vi "0926New Project.vi"() -> ()   [LabVIEW 2011] (continued)
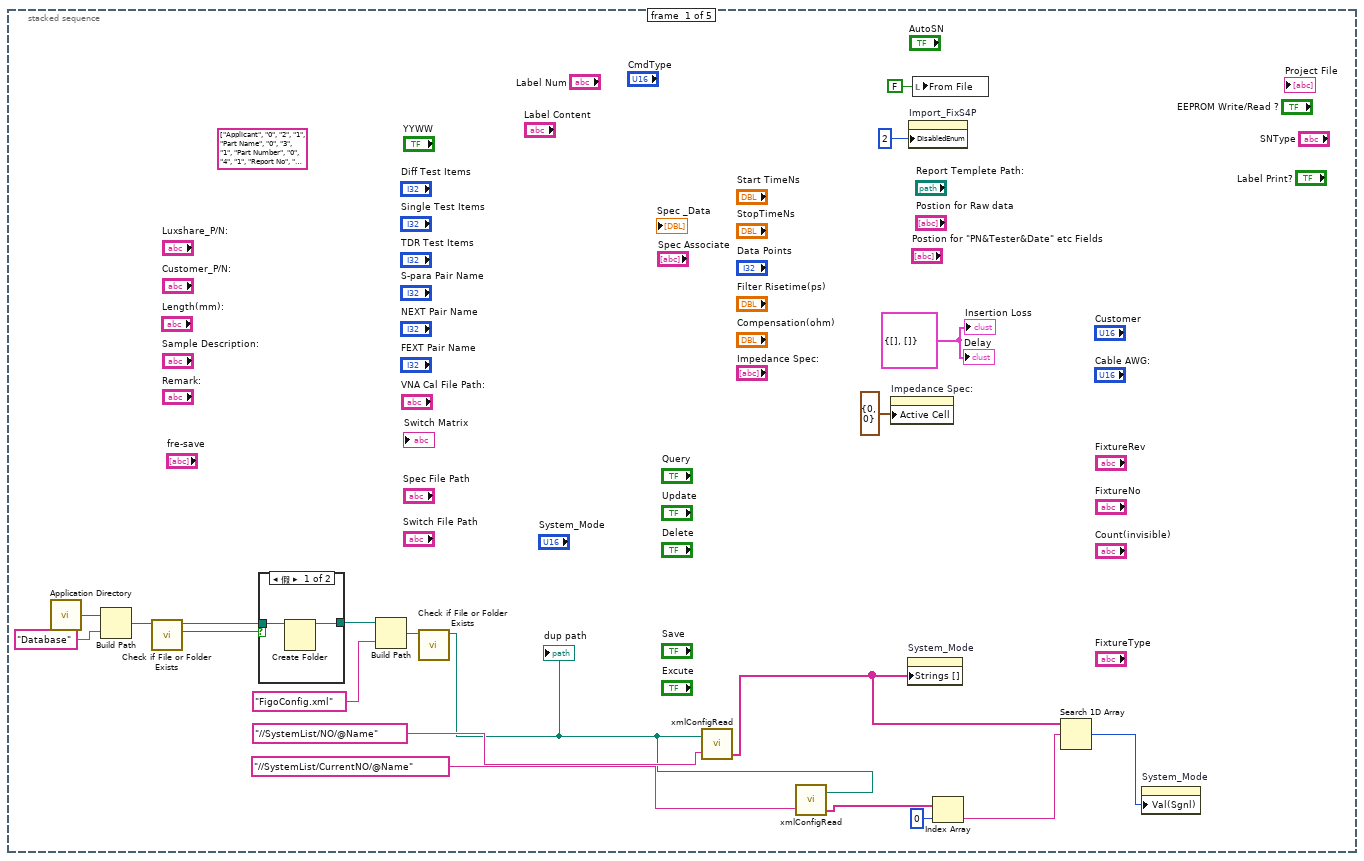
[diagram p3: hidden frame]
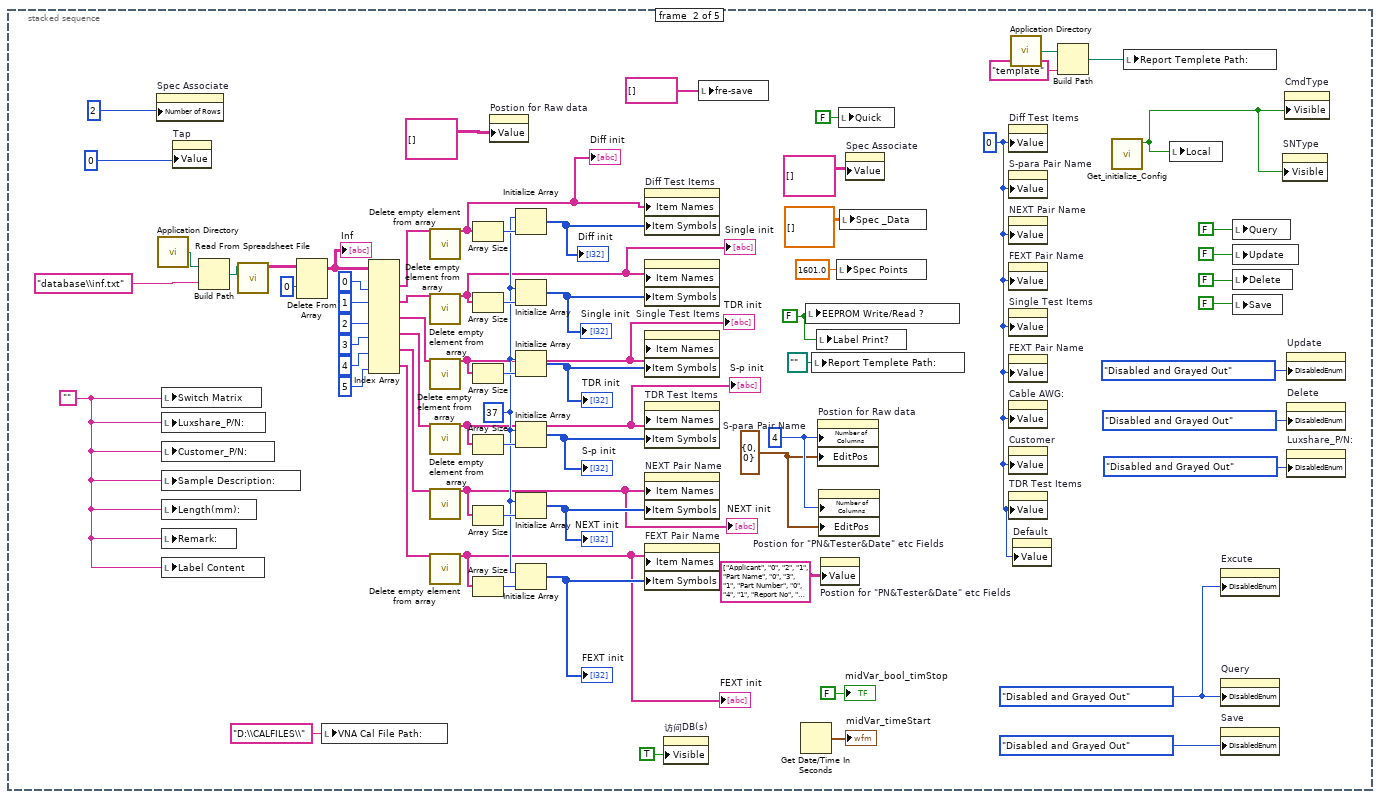
[diagram p5: hidden frame]
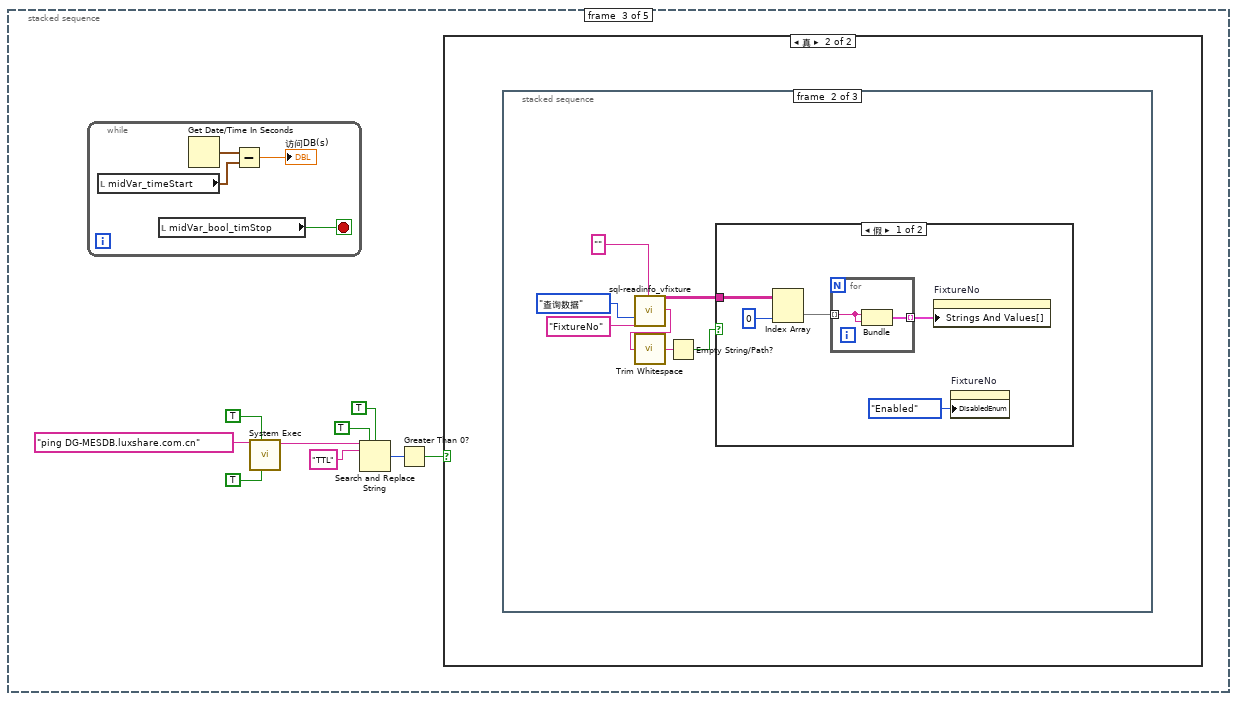
[diagram p6: hidden frame]
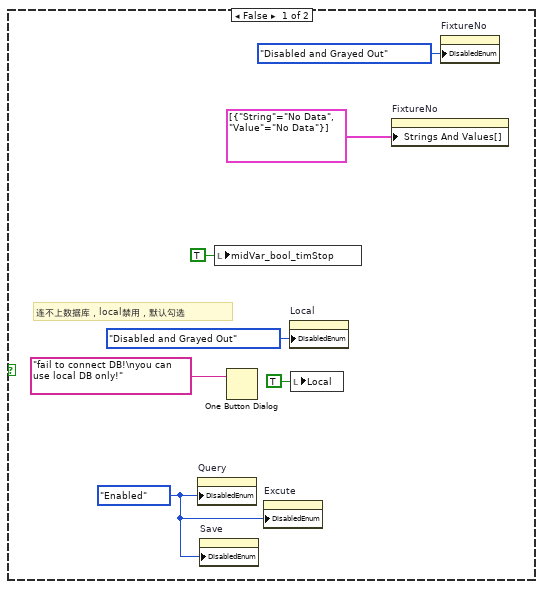
[diagram p7: hidden frame]
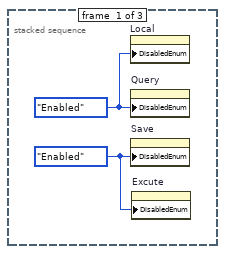
[diagram p8: hidden frame]
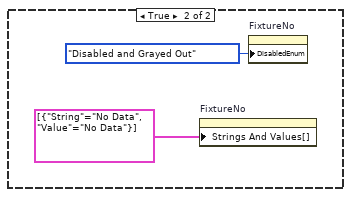
[diagram p9: hidden frame]
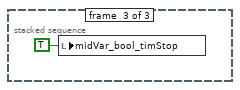
[diagram p10: hidden frame]
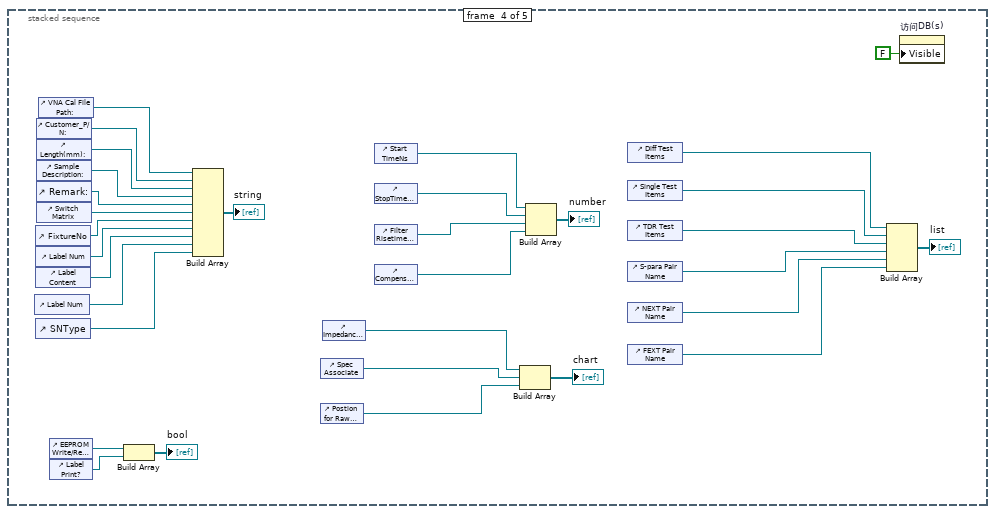
[diagram p11: hidden frame]
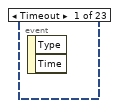
[diagram p12: hidden frame]
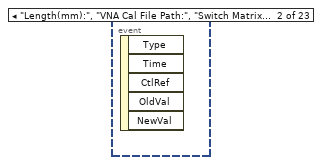
[diagram p13: hidden frame]
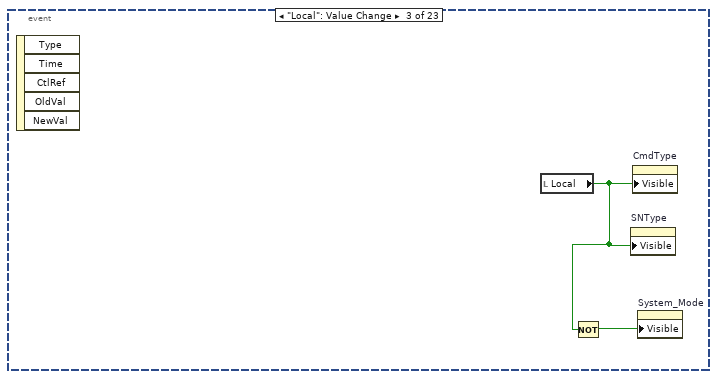
[diagram p14: hidden frame]
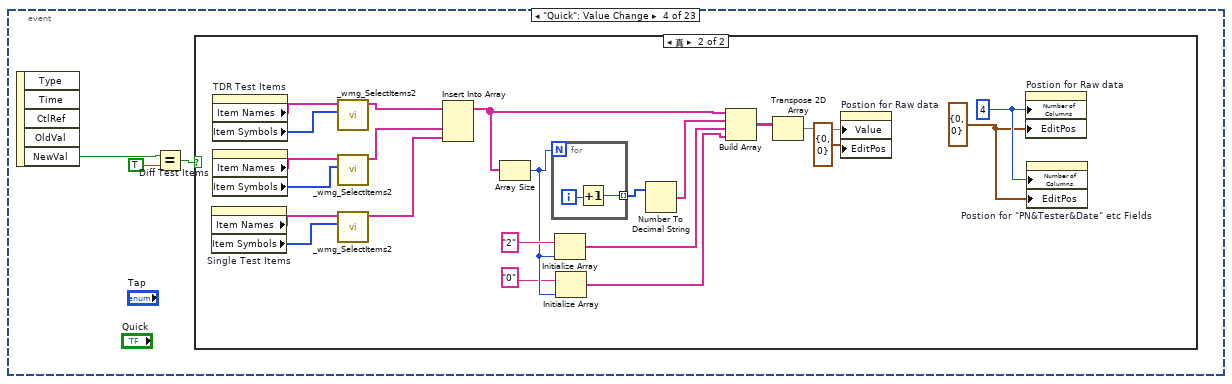
[diagram p15: hidden frame]
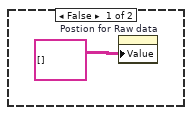
[diagram p16: hidden frame]
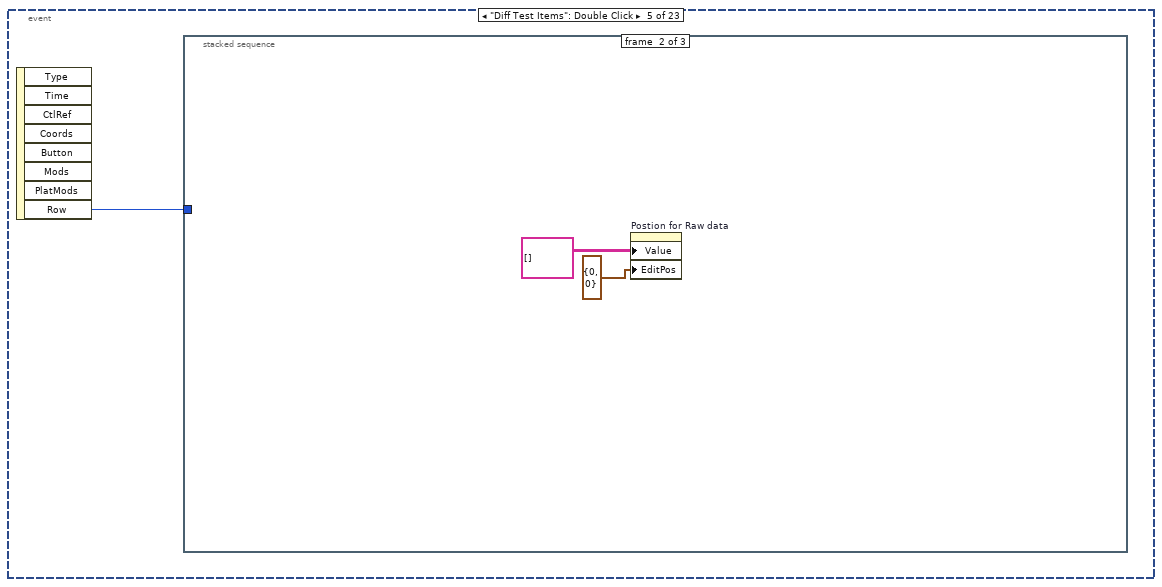
[diagram p17: hidden frame]
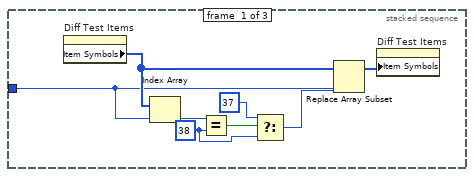
[diagram p18: hidden frame]
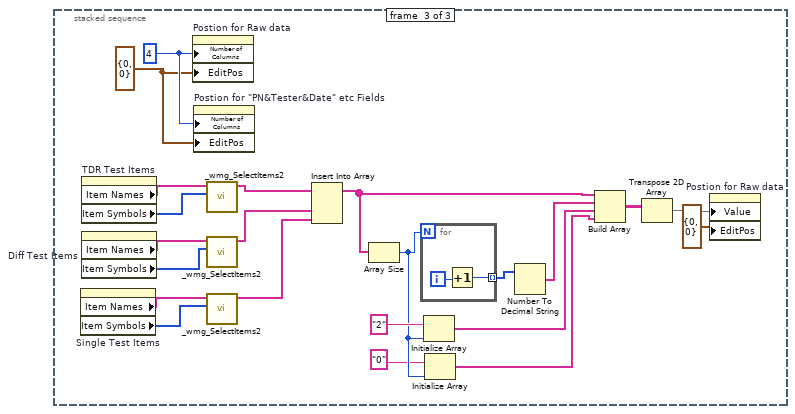
[diagram p19: hidden frame]
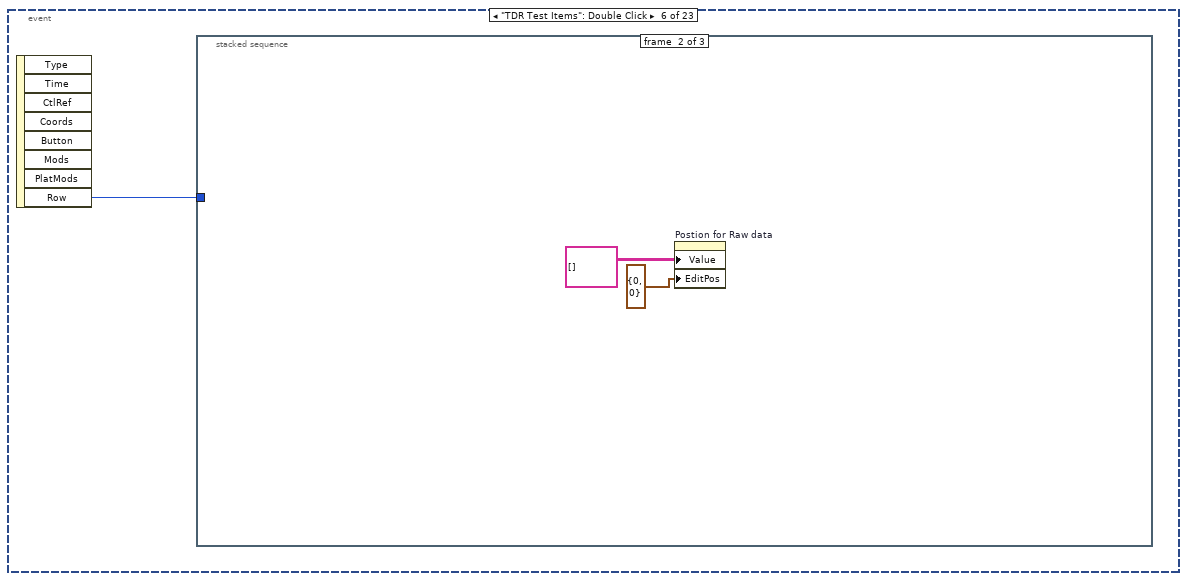
[diagram p20: hidden frame]
                    n969 = Number To Decimal String(number=w1171) -> (decimal integer string=w1169:string)  [unwired: 1 in]
                    n970 = call "impedance spec.vi"("Impedance Spec:"=w1168) -> ("Impedance spec string"=w1167:string)  [unwired: 10 in]
                    n971 = call <vilib>:"Trim Whitespace.vi"("string"=w1152) -> ("trimmed string"=w1144:string)  [unwired: 1 in]
                    n972 = Build Array(w1149, w1148, w1147, w1146, w1145, w1169, w1167, w1150, w1151, w1144) -> (→"TDR Setting":string[])
                    n973 = local read "Report Templete Path:"() -> (w1153:path)
                    n974 = property on="Postion for Raw data" class="Tbl (严格)"() -> ("Value"=w1165:string[][])  [unwired: 2 in, 2 out]
                    n975 = property on="Postion for \"PN&Tester&Date\" etc Fields" class="Tbl (严格)"() -> ("Value"=w1164:string[][])  [unwired: 2 in, 2 out]
                    n976 = Array To Spreadsheet String(array=w1165, 3:w1166) -> (spreadsheet string=w1161:string)  [unwired: 1 in]
                    n977 = Array To Spreadsheet String(array=w1164, 3:w1166) -> (spreadsheet string=w1159:string)  [unwired: 1 in]
                    n978 = Path To String(path=w1153) -> (string=w1154:string)
                    n979 = Search and Replace String(replace all?=TRUE ("替换全部？(F)"), input string=w1161, search string=w1156, replace string=w1155) -> (result string=w1158:string)  [unwired: 4 in, 3 out]
                    n980 = Search and Replace String(replace all?=TRUE ("替换全部？(F)"), input string=w1159, search string=w1156, replace string=w1155) -> (result string=w1157:string)  [unwired: 4 in, 3 out]
                    n981 = Build Array(w1154, w1158, w1157) -> (→"Report Config":string[])
                  }
                  frame #1 {
                    n982 = property on="S-para Pair Name" class="LstBox (严格)"() -> ("Item Names"=w1206:string[], "Item Symbols"=w1205:i32[])  [unwired: 2 in, 2 out]
                    n983 = property on="NEXT Pair Name" class="LstBox (严格)"() -> ("Item Names"=w1204:string[], "Item Symbols"=w1203:i32[])  [unwired: 2 in, 2 out]
                    n984 = property on="FEXT Pair Name" class="LstBox (严格)"() -> ("Item Names"=w1202:string[], "Item Symbols"=w1201:i32[])  [unwired: 2 in, 2 out]
                    n985 = local read "Spec Associate"() -> (w1195:string[][])
                    n986 = property on="Single Test Items" class="LstBox (严格)"() -> ("Item Names"=w1208:string[], "Item Symbols"=w1207:i32[])  [unwired: 2 in, 2 out]
                    n987 = property on="Diff Test Items" class="LstBox (严格)"() -> ("Item Names"=w1210:string[], "Item Symbols"=w1209:i32[])  [unwired: 2 in, 2 out]
                    n988 = property on="TDR Test Items" class="LstBox (严格)"() -> ("Item Names"=w1184:string[], "Item Symbols"=w1183:i32[])  [unwired: 2 in, 2 out]
                    n989 = call "Selected items.vi"("Item Syms"=w1205, "Item name"=w1206) -> ("Selected tem"=w1200:string[])  [unwired: 7 in, 2 out]
                    n990 = call "Selected items.vi"("Item Syms"=w1203, "Item name"=w1204) -> ("Selected tem"=w1199:string[])  [unwired: 7 in, 2 out]
                    n991 = call "Selected items.vi"("Item Syms"=w1201, "Item name"=w1202) -> ("Selected tem"=w1198:string[])  [unwired: 7 in, 2 out]
                    n992 = call "Selected items.vi"("Item Syms"=w1209, "Item name"=w1210) -> ("Selected tem"=w1197:string[])  [unwired: 7 in, 2 out]
                    n993 = call "Selected items.vi"("Item Syms"=w1207, "Item name"=w1208) -> ("Selected tem"=w1196:string[])  [unwired: 7 in, 2 out]
                    n994 = call "Selected items.vi"("Item Syms"=w1183, "Item name"=w1184) -> ("Selected tem"=w1181:string[])  [unwired: 7 in, 2 out]
                    n995 = Index Array(array=w1195, index (row)=1 ("索引 (行)")) -> (element=w1182:string[])  [unwired: 1 in]
                    n996 = local read "cancel dem2X?"() -> (w1176:bool)
                    n997 = local read "VNA Cal File Path:"() -> (w1178:string)
                    n998 = Select(t="TRUE", s=w1176, f="FALSE") -> (s? t:f=w1173:string)
                    n999 = local read "Report Config"() -> (w1179:string[])
                    n1000 = local read "TDR Setting"() -> (w1180:string[])
                    n1001 = Build Array(w1178) -> (w1193:string[])
                    n1002 = Number To Decimal String(number="ILD Spec") -> (decimal integer string=w1186:string)  [unwired: 1 in]
                    n1003 = Build Array(w1186) -> (w1185:string[])
                    n1004 = Build Array(w1173) -> (w1177:string[])
                    n1005 = Build Array(w1200, w1199, w1198, w1197, w1196, w1181, w1182, w1193, w1179, w1185, w1180, w1177) -> (w1192:string[][])
                    n1006 = Transpose 2D Array(2D array=w1192) -> (transposed array=w1191:string[][])
                    n1007 = Array To Spreadsheet String(delimiter (Tab)="#" ("分隔符(Tab)"), array=w1191, 3:"%s" ("格式字符串")) -> (spreadsheet string=→"Project Information":string)
                  }
                  frame #2 {
                    n1008 = local read "VNA Cal File Path:"() -> (w1230:string)
                    n1009 = property on="Diff Test Items" class="LstBox (严格)"() -> ("Item Symbols"=w1227:i32[])  [unwired: 2 in, 2 out]
                    n1010 = property on="Single Test Items" class="LstBox (严格)"() -> ("Item Symbols"=w1226:i32[])  [unwired: 2 in, 2 out]
                    n1011 = property on="TDR Test Items" class="LstBox (严格)"() -> ("Item Symbols"=w1225:i32[])  [unwired: 2 in, 2 out]
                    n1012 = property on="S-para Pair Name" class="LstBox (严格)"() -> ("Item Symbols"=w1224:i32[])  [unwired: 2 in, 2 out]
                    n1013 = property on="NEXT Pair Name" class="LstBox (严格)"() -> ("Item Symbols"=w1223:i32[])  [unwired: 2 in, 2 out]
                    n1014 = property on="FEXT Pair Name" class="LstBox (严格)"() -> ("Item Symbols"=w1219:i32[])  [unwired: 2 in, 2 out]
                    n1015 = local read "Luxshare_P/N:"() -> (w1217:string)
                    n1016 = local read "Length(mm):"() -> (w1231:string)
                    n1017 = String Length(string=w1217) -> (length=w1218:i32)
                    n1018 = Empty String/Path?(string/path=w1230) -> (empty?=w1228:bool)
                    n1019 = Empty String/Path?(string/path=w1231) -> (empty?=w1229:bool)
                    n1020 = Build Array(w1227, w1226, w1225, w1224, w1223, w1219) -> (w1222:i32[][])
                    n1021 = Not(x=w1229) -> (.not. x?=w1221:bool)
                    n1022 = Not(x=w1228) -> (.not. x?=w1220:bool)
                    n1023 = Greater Than 0?(x=w1218) -> (x > 0?=w1216:bool)
                    n1024 = call "_wmg_whetherItemsEmpty.vi"("Input"=w1222) -> ("bool"=w1232:bool)
                    n1025 = local read "Spec _Data"() -> (w1213:dbl[][])
                    n1026 = Compound Arithmetic op=AND(w1216, w1221, w1220, w1232) -> (→"save?":bool)
                    n1027 = Array To Spreadsheet String(delimiter (Tab)="#" ("分隔符(Tab)"), array=w1213, 3:"%s" ("格式字符串")) -> (spreadsheet string=w1214:string)
                    n1028 = local write "Spec String"(w1214) -> ()
                  }
                  frame #3 {
                    n1029 = local read "Local"() -> (w1233:bool)
                    n1030 = case shown="真" w1233 {
                      frame False {
                        # "16"
                        # "15"
                        # "14"
                        # "13"
                        # "11"
                        # "10"
                        # "9"
                        # "8"
                        # "7"
                        # "6"
                        # "5"
                        # "4"
                        # "3"
                        # "2"
                        # "1"
                        n1031 = local read "Label Print?"() -> (w1239:bool)
                        n1032 = local read "fre-save"() -> (w1246:string[])
                        n1033 = Boolean To (0,1)(Boolean=w1239) -> (0, 1=w1264:i16)
                        n1034 = local read "EEPROM Write/Read ?"() -> (w1240:bool)
                        n1035 = local read "Sample Description:"() -> (w1260:string)
                        n1036 = local read "Project Information"() -> (w1261:string)
                        n1037 = Array To Spreadsheet String(delimiter (Tab)="," ("分隔符(Tab)"), array=w1246, 3:"" ("格式字符串")) -> (spreadsheet string=w1243:string)
                        n1038 = Number To Decimal String(number=w1264) -> (decimal integer string=w1254:string)  [unwired: 1 in]
                        n1039 = local read "Customer_P/N:"() -> (w1263:string)
                        n1040 = local read "Switch Matrix"() -> (w1256:string)
                        n1041 = local read "Label Content"() -> (w1253:string)
                        n1042 = local read "Length(mm):"() -> (w1258:string)
                        n1043 = local read "Spec String"() -> (w1257:string)
                        n1044 = call <vilib>:"Trim Whitespace.vi"("string"=w1243) -> ("trimmed string"=w1242:string)  [unwired: 1 in]
                        n1045 = property on="Customer" class="Ring (严格)"() -> ("RingText.Text"=w1262:string)  [unwired: 2 in, 2 out]
                        n1046 = property on="Cable AWG:" class="Ring (严格)"() -> ("RingText.Text"=w1259:string)  [unwired: 2 in, 2 out]
                        n1047 = local read "FixtureNo"() -> (w1251:string)
                        n1048 = local read "Label Num"() -> (w1266:string)
                        n1049 = local read "Remark:"() -> (w1252:string)
                        n1050 = local read "Switch File Path"() -> (w1238:string)
                        n1051 = Boolean To (0,1)(Boolean=w1240) -> (0, 1=w1265:i16)
                        n1052 = local read "AutoSN"() -> (w1248:bool)
                        n1053 = Number To Decimal String(number=w1265) -> (decimal integer string=w1255:string)  [unwired: 1 in]
                        n1054 = Boolean To (0,1)(Boolean=w1248) -> (0, 1=w1249:i16)
                        n1055 = local read "Spec File Path"() -> (w1237:string)
                        n1056 = Number To Decimal String(number=w1249) -> (decimal integer string=w1247:string)  [unwired: 1 in]
                        n1057 = local read "Luxshare_P/N:"() -> (w1250:string)
                        n1058 = local read "Spec Points"() -> (w1236:dbl)
                        n1059 = property on="System_Mode" class="Ring (严格)"() -> ("RingText.Text"=w1234:string)  [unwired: 2 in, 2 out]
                        n1060 = Number To Decimal String(number=w1236) -> (decimal integer string=w1235:string)  [unwired: 1 in]
                        n1061 = Build Array(w1250, w1263, w1262, w1261, w1260, w1259, w1258, w1257, w1256, w1255, w1251, w1254, w1266, w1253, w1252, w1247, w1242, w1238, w1237, w1235, w1234) -> (w1241:string[])
                        n1062 = local write "Project File"(w1241) -> ()
                      }
                      frame True {
                        # "11"
                        # "10"
                        # "9"
                        # "8"
                        # "7"
                        # "6"
                        # "5"
                        # "4"
                        # "3"
                        # "2"
                        # "1"
                        n1063 = local read "Label Print?"() -> (w1272:bool)
                        n1064 = local read "fre-save"() -> (w1280:string[])
                        n1065 = Boolean To (0,1)(Boolean=w1272) -> (0, 1=w1299:i16)
                        n1066 = local read "EEPROM Write/Read ?"() -> (w1274:bool)
                        n1067 = property on="CmdType" class="Ring (严格)"() -> ("RingText.Text"=w1271:string)  [unwired: 2 in, 2 out]
                        n1068 = local read "Sample Description:"() -> (w1295:string)
                        n1069 = local read "Project Information"() -> (w1296:string)
                        n1070 = Array To Spreadsheet String(delimiter (Tab)="," ("分隔符(Tab)"), array=w1280, 3:"" ("格式字符串")) -> (spreadsheet string=w1277:string)
                        n1071 = local read "SNType"() -> (w1273:string)
                        n1072 = Number To Decimal String(number=w1299) -> (decimal integer string=w1289:string)  [unwired: 1 in]
                        n1073 = local read "Customer_P/N:"() -> (w1298:string)
                        n1074 = local read "Switch Matrix"() -> (w1291:string)
                        n1075 = local read "Label Content"() -> (w1288:string)
                        n1076 = local read "Length(mm):"() -> (w1293:string)
                        n1077 = local read "Spec String"() -> (w1292:string)
                        n1078 = call <vilib>:"Trim Whitespace.vi"("string"=w1277) -> ("trimmed string"=w1276:string)  [unwired: 1 in]
                        n1079 = property on="Customer" class="Ring (严格)"() -> ("RingText.Text"=w1297:string)  [unwired: 2 in, 2 out]
                        n1080 = property on="Cable AWG:" class="Ring (严格)"() -> ("RingText.Text"=w1294:string)  [unwired: 2 in, 2 out]
                        n1081 = local read "FixtureNo"() -> (w1286:string)
                        n1082 = local read "Label Num"() -> (w1301:string)
                        n1083 = local read "Remark:"() -> (w1287:string)
                        n1084 = call <vilib>:"Trim Whitespace.vi"("string"=w1271) -> ("trimmed string"=w1284:string)  [unwired: 1 in]
                        n1085 = local read "Switch File Path"() -> (w1270:string)
                        n1086 = Boolean To (0,1)(Boolean=w1274) -> (0, 1=w1300:i16)
                        n1087 = local read "AutoSN"() -> (w1282:bool)
                        n1088 = Number To Decimal String(number=w1300) -> (decimal integer string=w1290:string)  [unwired: 1 in]
                        n1089 = Boolean To (0,1)(Boolean=w1282) -> (0, 1=w1283:i16)
                        n1090 = Number To Decimal String(number=w1283) -> (decimal integer string=w1281:string)  [unwired: 1 in]
                        n1091 = local read "Luxshare_P/N:"() -> (w1285:string)
                        n1092 = local read "Spec File Path"() -> (w1269:string)
                        n1093 = local read "Spec Points"() -> (w1268:dbl)
                        n1094 = Number To Decimal String(number=w1268) -> (decimal integer string=w1267:string)  [unwired: 1 in]
                        n1095 = Build Array(w1285, w1298, w1297, w1296, w1295, w1294, w1293, w1292, w1291, w1290, w1284, w1273, w1286, w1289, w1301, w1288, w1287, w1281, w1276, w1270, w1269, w1267) -> (w1275:string[])
                        n1096 = local write "Project File"(w1275) -> ()
                      }
                    }
                  }
                  frame #4 {
                    n1097 = local read "save?"() -> (w1302:bool)
                    n1098 = case shown="真" w1302 {
                      frame False {
                        n1099 = One Button Dialog(message="保存信息不完整" ("消息")) -> ()  [unwired: 1 in, 1 out]
                      }
                      frame True {
                        n1100 = local read "Luxshare_P/N:"() -> (w1305:string)
                        n1101 = local read "Project File"() -> (w1304:string[])
                        n1102 = case shown="假" "Local" {
                          tunnel: w1304 -> [w1310 w1322]
                          tunnel: w1305 -> [_ w1330]
                          frame False {
                            # "保存至数据库"
                            n1103 = call "sql-writeinfo_vproject.vi"("操作模式"=enum16{"写入数据", "更改数据"}."写入数据", "列名"=string[] ["LuxsharePN", "CustomerPN", "Customer", "Prjinf", "SampleDes", "AWG", "Length", "Spec", "SwitchMatrix", "EEPROMTF", "FixtureNo", "LabelTF", "LabelNum", "LabelC", "Remark", "AutoSN", "FrePoints", "Switch_File_Path", "Spec_File_Path", "Spec_Points", "HardWare_Mode"], "值"=w1310) -> ("简单报错"=w1308:string, "status"=w1309:bool)  [unwired: 15 in]
                            n1104 = case shown="真" w1309 {
                              tunnel: w1308 -> [_ w1321]
                              frame False {
                                # "清空操作"
                                n1105 = control-ref of="Report Templete Path:"() -> (w1315:refnum<vi>)
                                n1106 = control-ref of="Data Points"() -> (w1314:refnum<vi>)
                                n1107 = control-ref of="Spec _Data"() -> (w1313:refnum<vi>)
                                n1108 = local read "bool"() -> (w1312:refnum<vi>[])
                                n1109 = One Button Dialog(message="Save Finished!" ("消息")) -> ()  [unwired: 1 in, 1 out]
                                n1110 = local read "number"() -> (w1316:refnum<vi>[])
                                n1111 = local read "string"() -> (w1319:refnum<vi>[])
                                n1112 = local read "chart"() -> (w1317:refnum<vi>[])
                                n1113 = local read "list"() -> (w1318:refnum<vi>[])
                                n1114 = call "_wmg_initAllCtrls.vi"("chart"=w1317, "number"=w1316, "list"=w1318, "string"=w1319, "bool"=w1312, "Spec _Data"=w1313, "Data Points"=w1314, "Report Templete Path:"=w1315) -> ()
                              }
                              frame True {
                                n1115 = One Button Dialog(message=w1321) -> ()  [unwired: 1 in, 1 out]
                              }
                            }
                          }
                          frame True {
                            n1116 = call <vilib>:"Application Directory.vi"() -> ("Application Directory"=w1329:path)
                            n1117 = Concatenate Strings("Database\\" ("字符串"), w1330, ".hpj" ("字符串")) -> (w1328:string)
                            n1118 = Build Path(base path=w1329, name or relative path=w1328) -> (appended path=w1325:path)
                            n1119 = call <vilib>:"Check if File or Folder Exists.vi"("path"=w1325) -> ("file or folder exists?"=w1324:bool, "dup path"=w1323:path)  [unwired: 8 in, 1 out]
                            n1120 = case shown="假" w1324 {
                              tunnel: w1323 -> [w1333 w1344]
                              tunnel: w1322 -> [w1332 w1343]
                              frame False {
                                # "清空操作"
                                n1121 = One Button Dialog(message="Local file save Finished!" ("消息")) -> ()  [unwired: 1 in, 1 out]
                                n1122 = control-ref of="Report Templete Path:"() -> (w1339:refnum<vi>)
                                n1123 = control-ref of="Data Points"() -> (w1340:refnum<vi>)
                                n1124 = control-ref of="Spec _Data"() -> (w1341:refnum<vi>)
                                n1125 = local read "bool"() -> (w1331:refnum<vi>[])
                                n1126 = Write to Binary File(file (use dialog)=w1333, data=w1332, 9:T7."big-endian, network order" ("字节顺序(0:big-endian, network order)")) -> ()  [unwired: 3 in, 3 out]
                                n1127 = local read "number"() -> (w1338:refnum<vi>[])
                                n1128 = local read "string"() -> (w1335:refnum<vi>[])
                                n1129 = local read "chart"() -> (w1337:refnum<vi>[])
                                n1130 = local read "list"() -> (w1336:refnum<vi>[])
                                n1131 = call "_wmg_initAllCtrls.vi"("chart"=w1337, "number"=w1338, "list"=w1336, "string"=w1335, "bool"=w1331, "Spec _Data"=w1341, "Data Points"=w1340, "Report Templete Path:"=w1339) -> ()
                              }
                              frame True {
                                n1132 = Two Button Dialog(message="该PN的文件已经存在\n是否覆盖？", 1:"取消" ("F按钮名称（“取消”）"), 2:"覆盖" ("T按钮名称（“确定”）")) -> (T button?=w1345:bool)
                                n1133 = case shown="真" w1345 {
                                tunnel: w1344 -> [_ w1350]
                                tunnel: w1343 -> [_ w1349]
                                frame False {
                                }
                                frame True {
                                n1134 = stacked-sequence {
                                tunnel: w1350 -> [w1353 _]
                                tunnel: w1349 -> [w1351 _]
                                frame #0 {
                                n1135 = One Button Dialog(message="Coved successfully!" ("消息")) -> ()  [unwired: 1 in, 1 out]
                                n1136 = Write to Binary File(file (use dialog)=w1353, data=w1351, 9:T7."big-endian, network order" ("字节顺序(0:big-endian, network order)")) -> ()  [unwired: 3 in, 3 out]
                                }
                                frame #1 {
                                # "清空操作"
                                n1137 = control-ref of="Report Templete Path:"() -> (w1359:refnum<vi>)
                                n1138 = control-ref of="Data Points"() -> (w1360:refnum<vi>)
                                n1139 = control-ref of="Spec _Data"() -> (w1361:refnum<vi>)
                                n1140 = local read "number"() -> (w1358:refnum<vi>[])
                                n1141 = local read "string"() -> (w1355:refnum<vi>[])
                                n1142 = local read "chart"() -> (w1357:refnum<vi>[])
                                n1143 = local read "list"() -> (w1356:refnum<vi>[])
                                n1144 = call "_wmg_initAllCtrls.vi"("chart"=w1357, "number"=w1358, "list"=w1356, "string"=w1355, "Spec _Data"=w1361, "Data Points"=w1360, "Report Templete Path:"=w1359) -> ()  [unwired: 1 in]
                                }
                                }
                                }
                                }
                              }
                            }
                          }
                        }
                      }
                    }
                  }
                  frame #5 {
                    w1362 = u16 0 items=["", "Common", "H3C psw 10G", "H3C psw 28G"] ("CmdType")
                    n1145 = property on="Update" class="Bool (严格)"("DisabledEnum"=T4."Disabled and Grayed Out" ("禁用")) -> ()  [unwired: 2 in, 2 out]
                    n1146 = property on="Delete" class="Bool (严格)"("DisabledEnum"=T4."Disabled and Grayed Out" ("禁用")) -> ()  [unwired: 2 in, 2 out]
                    n1147 = property on="Luxshare_P/N:" class="Str"("DisabledEnum"=T4."Disabled and Grayed Out" ("禁用")) -> ()  [unwired: 2 in, 2 out]
                    n1148 = local write "CmdType"(w1362) -> ()
                    n1149 = local write "Query"(FALSE ("Query")) -> ()
                    n1150 = local write "Update"(FALSE ("Query")) -> ()
                    n1151 = local write "Delete"(FALSE ("Query")) -> ()
                    n1152 = local write "Save"(FALSE ("Query")) -> ()
                  }
                }
              }
            }
          }
          event "System_Mode": Value Change {
            w1374 = "@NameVar@" ("搜索字符串")
            n1153 = event-data() -> ("NewVal"=w1383:u16)  [unwired: 1 in, 4 out]
            n1154 = property on="System_Mode" class="Ring (严格)"() -> ("Strings []"=w1384:string[])  [unwired: 2 in, 2 out]
            n1155 = local read "dup path"() -> (w1377:path)
            n1156 = Index Array(array=w1384, index=w1383) -> (element=w1370:string)
            n1157 = Search and Replace String(input string="//SystemList/NO[@Name='@NameVar@']/@Switch" ("XPath expression"), search string=w1374, replace string=w1370) -> (result string=w1381:string)  [unwired: 5 in, 3 out]
            n1158 = call "xmlConfigRead.vi"("path to XML document"=w1377, "XPath expression"=w1381) -> ("OutParaArray"=w1380:string[])  [unwired: 2 out]
            n1159 = Index Array(array=w1380, index=0 ("索引")) -> (element=→"开关型号":string)
            n1160 = Search and Replace String(input string="//SystemList/NO[@Name='@NameVar@']/@Equipment" ("XPath expression"), search string=w1374, replace string=w1370) -> (result string=w1376:string)  [unwired: 5 in, 3 out]
            n1161 = call "xmlConfigRead.vi"("path to XML document"=w1377, "XPath expression"=w1376) -> ("OutParaArray"=w1373:string[])  [unwired: 2 out]
            n1162 = Index Array(array=w1373, index=0 ("索引")) -> (element=→"仪器型号":string)
          }
          event Panel Close {
            n1163 = event-data() -> ()  [unwired: 1 in, 3 out]
          }
          event "Default": Value Change {
            n1164 = event-data() -> ()  [unwired: 1 in, 5 out]
            n1165 = case shown="\"Default\", 默认" "Default" {
              frame "Default", Default {
                w1387 = 0 ("Diff Test Items")
                w1393 = 37
                n1166 = local read "Inf"() -> (w1412:string[][])
                n1167 = Index Array(array=w1412, index (col) #1=0 ("禁用的索引 (列)"), index (col) #2=1 ("索引 (列)"), index (col) #3=2 ("索引 (列)"), index (col) #4=3 ("索引 (列)"), index (col) #5=4 ("索引 (列)"), index (col) #6=5 ("索引 (列)")) -> (element #1=w1406:string[], element #2=w1405:string[], element #3=w1404:string[], element #4=w1403:string[], element #5=w1402:string[], element #6=w1396:string[])  [unwired: 6 in]
                n1168 = call "Delete empty element from array.vi"("Array In"=w1396) -> ("Array out"=w1388:string[])  [unwired: 26 in]
                n1169 = call "Delete empty element from array.vi"("Array In"=w1406) -> ("Array out"=w1397:string[])  [unwired: 26 in]
                n1170 = call "Delete empty element from array.vi"("Array In"=w1402) -> ("Array out"=w1389:string[])  [unwired: 26 in]
                n1171 = call "Delete empty element from array.vi"("Array In"=w1405) -> ("Array out"=w1398:string[])  [unwired: 26 in]
                n1172 = call "Delete empty element from array.vi"("Array In"=w1404) -> ("Array out"=w1391:string[])  [unwired: 26 in]
                n1173 = call "Delete empty element from array.vi"("Array In"=w1403) -> ("Array out"=w1390:string[])  [unwired: 26 in]
                n1174 = Array Size(array=w1397) -> (size(s)=w1419:i32)
                n1175 = Array Size(array=w1398) -> (size(s)=w1413:i32)
                n1176 = Array Size(array=w1391) -> (size(s)=w1392:i32)
                n1177 = Array Size(array=w1390) -> (size(s)=w1399:i32)
                n1178 = Array Size(array=w1389) -> (size(s)=w1416:i32)
                n1179 = Array Size(array=w1388) -> (size(s)=w1400:i32)
                n1180 = Initialize Array(w1393, w1419) -> (w1418:i32[])
                n1181 = Initialize Array(w1393, w1413) -> (w1414:i32[])
                n1182 = Initialize Array(w1393, w1399) -> (w1417:i32[])
                n1183 = Initialize Array(w1393, w1392) -> (w1394:i32[])
                n1184 = Initialize Array(w1393, w1416) -> (w1415:i32[])
                n1185 = Initialize Array(w1393, w1400) -> (w1401:i32[])
                n1186 = property on="Diff Test Items" class="LstBox (严格)"("Item Names"=w1397, "Item Symbols"=w1418) -> ()  [unwired: 2 in, 2 out]
                n1187 = property on="Single Test Items" class="LstBox (严格)"("Item Names"=w1398, "Item Symbols"=w1414) -> ()  [unwired: 2 in, 2 out]
                n1188 = property on="TDR Test Items" class="LstBox (严格)"("Item Names"=w1391, "Item Symbols"=w1394) -> ()  [unwired: 2 in, 2 out]
                n1189 = property on="S-para Pair Name" class="LstBox (严格)"("Item Names"=w1390, "Item Symbols"=w1417) -> ()  [unwired: 2 in, 2 out]
                n1190 = property on="NEXT Pair Name" class="LstBox (严格)"("Item Names"=w1389, "Item Symbols"=w1415) -> ()  [unwired: 2 in, 2 out]
                n1191 = property on="FEXT Pair Name" class="LstBox (严格)"("Item Names"=w1388, "Item Symbols"=w1401) -> ()  [unwired: 2 in, 2 out]
                n1192 = property on="Diff Test Items" class="LstBox (严格)"("Value"=w1387, "Top Row"=w1387) -> ()  [unwired: 2 in, 2 out]
                n1193 = property on="Single Test Items" class="LstBox (严格)"("Value"=w1387, "Top Row"=w1387) -> ()  [unwired: 2 in, 2 out]
                n1194 = property on="TDR Test Items" class="LstBox (严格)"("Value"=w1387, "Top Row"=w1387) -> ()  [unwired: 2 in, 2 out]
                n1195 = property on="S-para Pair Name" class="LstBox (严格)"("Value"=w1387, "Top Row"=w1387) -> ()  [unwired: 2 in, 2 out]
                n1196 = property on="NEXT Pair Name" class="LstBox (严格)"("Value"=w1387, "Top Row"=w1387) -> ()  [unwired: 2 in, 2 out]
                n1197 = property on="FEXT Pair Name" class="LstBox (严格)"("Value"=w1387, "Top Row"=w1387) -> ()  [unwired: 2 in, 2 out]
              }
              frame "Quick" {
                w1420 = 0 ("Diff Test Items")
                w1424 = 38
                n1198 = local read "Inf"() -> (w1442:string[][])
                n1199 = Index Array(array=w1442, index (col) #1=0 ("禁用的索引 (列)"), index (col) #2=1 ("索引 (列)"), index (col) #3=3 ("索引 (列)"), index (col) #4=4 ("索引 (列)"), index (col) #5=5 ("索引 (列)")) -> (element #1=w1436:string[], element #2=w1435:string[], element #3=w1434:string[], element #4=w1433:string[], element #5=w1432:string[])  [unwired: 5 in]
                n1200 = call "Delete empty element from array.vi"("Array In"=w1436) -> ("Array out"=w1425:string[])  [unwired: 26 in]
                n1201 = call "Delete empty element from array.vi"("Array In"=w1432) -> ("Array out"=w1429:string[])  [unwired: 26 in]
                n1202 = call "Delete empty element from array.vi"("Array In"=w1435) -> ("Array out"=w1426:string[])  [unwired: 26 in]
                n1203 = call "Delete empty element from array.vi"("Array In"=w1434) -> ("Array out"=w1427:string[])  [unwired: 26 in]
                n1204 = call "Delete empty element from array.vi"("Array In"=w1433) -> ("Array out"=w1428:string[])  [unwired: 26 in]
                n1205 = Array Size(array=w1426) -> (size(s)=w1443:i32)
                n1206 = Array Size(array=w1428) -> (size(s)=w1446:i32)
                n1207 = Array Size(array=w1429) -> (size(s)=w1430:i32)
                n1208 = Initialize Array(37, w1443) -> (w1444:i32[])
                n1209 = Initialize Array(w1424, w1446) -> (w1445:i32[])
                n1210 = Initialize Array(w1424, w1430) -> (w1431:i32[])
                n1211 = property on="Diff Test Items" class="LstBox (严格)"("Item Names"=w1425, "Item Symbols"=i32[] [38, 37, 37, 38, 38, 37, 38, 37, 37, 37, 37, 37, 37, 37, 37, 37, 37, 37, 38, 38] ("初始化的数组")) -> ()  [unwired: 2 in, 2 out]
                n1212 = property on="Single Test Items" class="LstBox (严格)"("Item Names"=w1426, "Item Symbols"=w1444) -> ()  [unwired: 2 in, 2 out]
                n1213 = property on="S-para Pair Name" class="LstBox (严格)"("Item Names"=w1427, "Item Symbols"=i32[] [38, 38, 38, 38, 38, 38, 38, 38, 37, 37, 37, 37, 37, 37, 37, 37] ("初始化的数组")) -> ()  [unwired: 2 in, 2 out]
                n1214 = property on="NEXT Pair Name" class="LstBox (严格)"("Item Names"=w1428, "Item Symbols"=w1445) -> ()  [unwired: 2 in, 2 out]
                n1215 = property on="FEXT Pair Name" class="LstBox (严格)"("Item Names"=w1429, "Item Symbols"=w1431) -> ()  [unwired: 2 in, 2 out]
                n1216 = property on="Diff Test Items" class="LstBox (严格)"("Value"=w1420, "Top Row"=w1420) -> ()  [unwired: 2 in, 2 out]
                n1217 = property on="Single Test Items" class="LstBox (严格)"("Value"=w1420, "Top Row"=w1420) -> ()  [unwired: 2 in, 2 out]
                n1218 = property on="TDR Test Items" class="LstBox (严格)"("Value"=w1420, "Top Row"=w1420) -> ()  [unwired: 2 in, 2 out]
                n1219 = property on="NEXT Pair Name" class="LstBox (严格)"("Value"=w1420, "Top Row"=w1420) -> ()  [unwired: 2 in, 2 out]
                n1220 = property on="FEXT Pair Name" class="LstBox (严格)"("Value"=w1420, "Top Row"=w1420) -> ()  [unwired: 2 in, 2 out]
                n1221 = property on="S-para Pair Name" class="LstBox (严格)"("Value"=w1420, "Top Row"=w1420) -> ()  [unwired: 2 in, 2 out]
              }
            }
          }
          event "Default  fre": Value Change {
            n1222 = event-data() -> ()  [unwired: 1 in, 5 out]
            n1223 = case shown="\"Clear\"" "Default  fre" {
              frame "Default", Default {
                n1224 = local write "fre-save"(string[] ["2500", "4500", "5000", "5156.25", "6000", "9000", "10000", "12890", "19000", "20000"]) -> ()
              }
              frame "Clear" {
                n1225 = local write "fre-save"(string[] [] ("fre-save")) -> ()
              }
            }
          }
          event "Default": Value Change {
            n1226 = event-data() -> ()  [unwired: 1 in, 5 out]
            n1227 = case shown="真" "Default" {
              frame False {
              }
              frame True {
                n1228 = property on="Postion for \"PN&Tester&Date\" etc Fields" class="Tbl (严格)"("Value"=string[][] [["Applicant", "0", "2", "1"], ["Part Name", "0", "3", "1"], ["Part Number", "0", "4", "1"], ["Report No", "0", "2", "12"], ["Sample No", "0", "4", "12"], ["Prepared By", "0", "63", "0"], ["Approved By", "0", "63", "6"], ["Date", "0", "63", "2"], ["Thru Result", "0", "13", "5"], ["NEXT Result", "0", "45", "4"], ["FEXT Result", "0", "45", "5"]] ("Postion for \"PN&Tester&Date\" etc Fields"), "Active Cell"=T3 {"Row"=0, "Column"=0} ("编辑位置")) -> ()  [unwired: 2 in, 2 out]
              }
            }
          }
        }
      }
    }
  }
  n1229 = disable-structure shown="禁用" {
    frame Disabled {
      n1230 = local read "Switch File Path"() -> ()  [unwired: 1 out]
      n1231 = local read "Spec File Path"() -> ()  [unwired: 1 out]
      n1232 = local read "Spec Points"() -> ()  [unwired: 1 out]
      n1233 = Number To Decimal String() -> ()  [unwired: 2 in, 1 out]
    }
    frame Enabled {
    }
  }
